vi "Set Destination.vi"(8 "error in (no error)":errorcluster, 9 "Destination label":string, 10 "ProjectItem Refnum":refnum<vi>, 11 "Build in":refnum<class "NI_AB_API_RESTful.lvclass">) -> (0 "error out":errorcluster, 3 "Build out":refnum<class "NI_AB_API_RESTful.lvclass">)   [LabVIEW 2020, in "NI_AB_API_RESTful.lvclass"]
uses:
  <vilib>/AppBuilder/AB_API/RESTful/NI_AB_API_RESTful.lvclass
  <vilib>/AppBuilder/AB_API/RESTful/NI_AB_API_RESTful.lvclass/NI_AB_API_RESTful.ctl
  <vilib>/AppBuilder/AB_API/Targetfile/NI_AB_API_Targetfile.lvclass
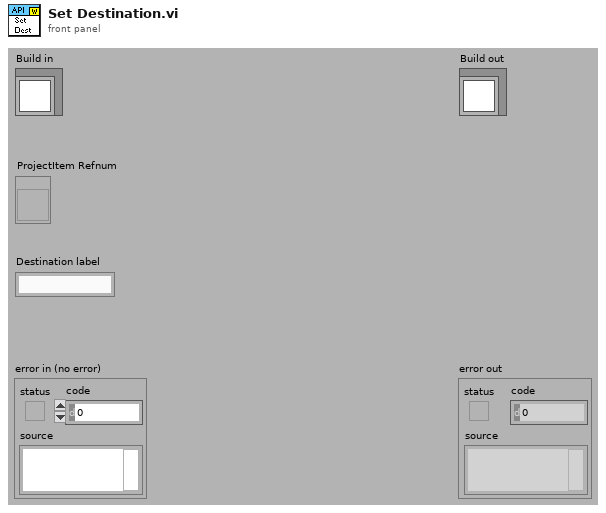
[diagram p1: front panel]
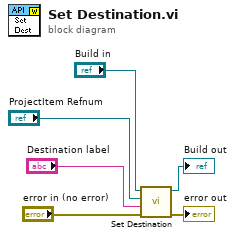
[diagram p0: block diagram]
diagram:
  n1 = call-parent "Set Destination.vi"("error in (no error)"="error in (no error)", "Destination label"="Destination label", "ProjectItem Refnum"="ProjectItem Refnum", "Build in"="Build in") -> ("error out"=→"error out":errorcluster, "Build out"=→"Build out":refnum<class "NI_AB_API_RESTful.lvclass">)  [unwired: 6 in]
